vi "getValueFromXMLNative.vi"(8 "error in (no error)":errorcluster, 10 "eventXML":refnum<k20>, 11 "RampEvent in":refnum<class "RampEvent.lvclass">) -> (0 "error out":errorcluster, 2 "eventXML out":refnum<k20>, 3 "RampEvent out":refnum<class "RampEvent.lvclass">)   [LabVIEW 2009, in "Tools.lvlib" / "Scripting.lvlib" / "RampEvent.lvclass"]
uses:
  RampEvent.lvclass
  <vilib>/xml/Close Reference(Node).vi
  <vilib>/xml/NI_XML.lvlib
  ScriptEvent.lvclass
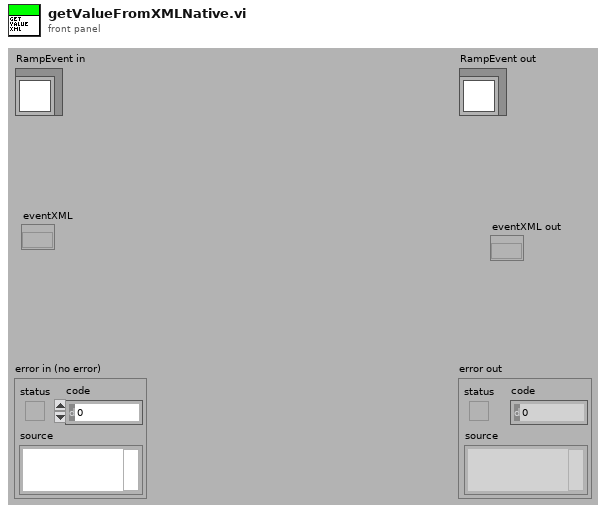
[diagram p1: front panel]
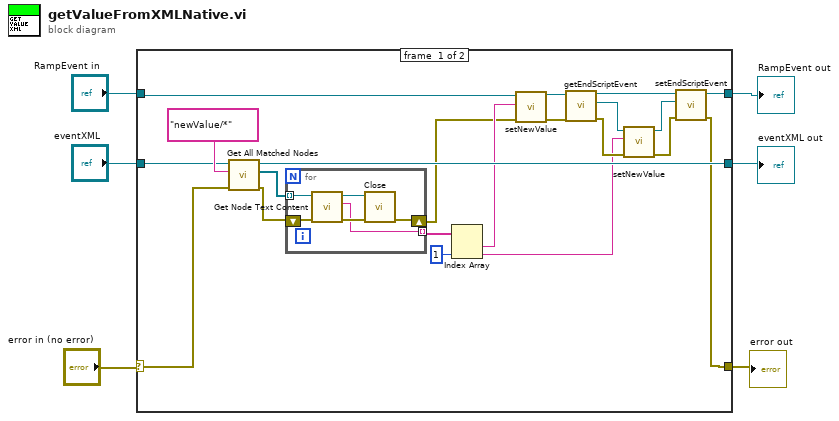
[diagram p0: block diagram]
diagram:
  n1 = case shown="No Error" "error in (no error)" {
    selector: "error in (no error)" -> [w8 w34]
    tunnel: [w7 w34] -> w5
    tunnel: [w16 w35] -> w4
    tunnel: "RampEvent in" -> [w17 w35]
    tunnel: "eventXML" -> [w25 _]
    tunnel: [w23 _] -> w1
    frame #0 {
      n2 = call <vilib>:"Get All Matched Nodes.vi"("error in (no error)"=w8, "XPath expression"="newValue/*", "node in"=w25) -> ("error out"=w27:errorcluster, "node result array"=w24:refnum<k20>[], "node out"=w23:refnum<k20>)  [unwired: 6 in]
      n3 = for {
        tunnel: w24 -> [w30] mode=indexing
        tunnel: [w29] -> w13 mode=indexing
        shift-right: [w28] -> w9
        shift-left: w27 -> [w31]
        n4 = call <vilib>:"Get Node Text Content.vi"("error in (no error)"=w31, "node in"=w30) -> ("error out"=w32:errorcluster, "node text"=w29:string, "node out"=w33:refnum<k20>)  [unwired: 7 in]
        n5 = call-poly <vilib>:"Close.vi"("error in (no error)"=w32, "node"=w33) -> ("error out"=w28:errorcluster)  [unwired: 7 in]
      }
      n6 = Index Array(array=w13, index #2=1 ("index")) -> (element #1=w12:string, element #2=w11:string)  [unwired: 1 in]
      n7 = call "setNewValue.vi"("error in (no error)"=w9, "newValue"=w12, "ScriptEvent.lvclass in"=w17) -> ("error out"=w21:errorcluster, "ScriptEvent.lvclass out"=w22:refnum<class "RampEvent.lvclass">)  [unwired: 7 in]
      n8 = call "getEndScriptEvent.vi"("error in (no error)"=w21, "RampEvent.lvclass in"=w22) -> ("error out"=w14:errorcluster, "ScriptEvent.lvclass"=w20:refnum<class "ScriptEvent.lvclass">, "RampEvent.lvclass out"=w18:refnum<class "RampEvent.lvclass">)  [unwired: 7 in]
      n9 = call "setNewValue.vi"("error in (no error)"=w14, "newValue"=w11, "ScriptEvent.lvclass in"=w20) -> ("error out"=w15:errorcluster, "ScriptEvent.lvclass out"=w19:refnum<class "ScriptEvent.lvclass">)  [unwired: 7 in]
      n10 = call "setEndScriptEvent.vi"("error in (no error)"=w15, "endScriptEvent.lvclass"=w19, "RampEvent.lvclass in"=w18) -> ("error out"=w7:errorcluster, "RampEvent.lvclass out"=w16:refnum<class "RampEvent.lvclass">)  [unwired: 7 in]
    }
    frame #1 {
    }
  }
  "error out" <- w5
  "RampEvent out" <- w4
  "eventXML out" <- w1
